vi "Keithley 6514 Setup Zero Correct.vi"(0 "Resource In":refnum<visa-resource-name>, 1 "Check For SCPI Errors? (T)":bool=TRUE, 7 "Zero Correct (Off:F)":bool, 9 "Acquire New Zero Correct Value? (No:F)":bool, 11 "error in (no error)":T1) -> (4 "Resource Out (dupl)":refnum<visa-resource-name>, 15 "error out":T1)   [LabVIEW 2014, in "KE6514Driver.lvlib"]
doc: "This VI for the Keithley 6514 Electrometer allows the operator to turn the 'Zero Correct' function on or off.\n\nZero Correct:\n1 or True: Zero Check On\n0 or False: Zero Check Off\n\nAcquire New Zero Correct Value\n1 or True: YES\n0 or False: NO"
uses:
  KE6514Driver.lvlib
panel:
  # "ON\nOFF"
  # "YES\nNO"
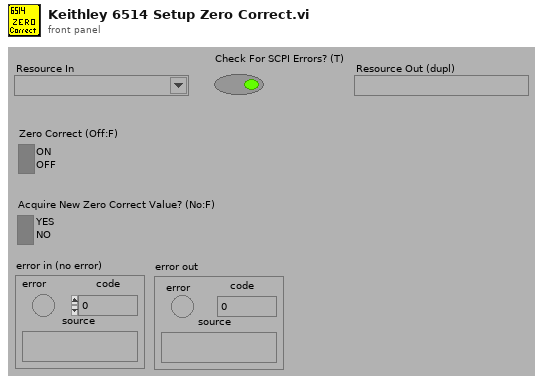
[diagram p1: front panel]
types:
  T1 = cluster{"error":bool, "code":i32, "source":string}
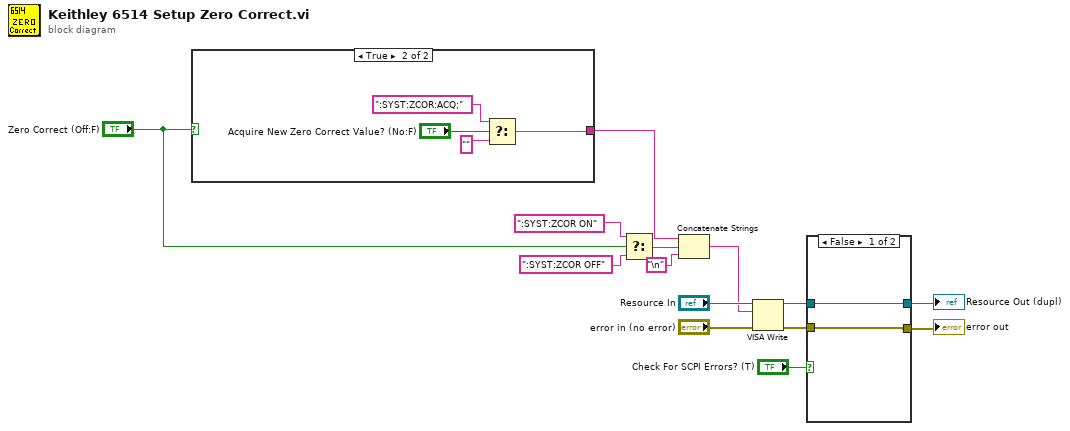
[diagram p0: block diagram]
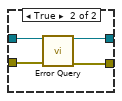
[diagram p2: hidden frame]
diagram:
  n1 = case shown="True" "Zero Correct (Off:F)" {
    tunnel: [_ w15] -> w11
    frame False {
    }
    frame True {
      n2 = Select(t=":SYST:ZCOR:ACQ;", s="Acquire New Zero Correct Value? (No:F)", f="") -> (s? t:f=w15:string)
    }
  }
  n3 = Select(t=":SYST:ZCOR ON", s="Zero Correct (Off:F)", f=":SYST:ZCOR OFF") -> (s? t:f=w10:string)
  n4 = Concatenate Strings(w11, w10, "\n") -> (w7:string)
  n5 = VISA Write(VISA resource name="Resource In", write buffer=w7, error in (no error)="error in (no error)") -> (VISA resource name out=w4:refnum<visa-resource-name>, error out=w3:errorcluster)  [unwired: 1 out]
  n6 = case shown="False" "Check For SCPI Errors? (T)" {
    tunnel: w4 -> [w20 w24]
    tunnel: w3 -> [w19 w23]
    tunnel: [w19 w22] -> w1
    tunnel: [w20 w21] -> w2
    frame False {
    }
    frame True {
      n7 = call "Error Query.vi"("VISA Resource In"=w24, "error in (no error)"=w23) -> ("VISA Resource Out (dupl)"=w21:refnum<visa-resource-name>, "error out"=w22:errorcluster)  [unwired: 10 in, 2 out]
    }
  }
  "error out" <- w1
  "Resource Out (dupl)" <- w2
